vi "read numarray, compare with original one.vi"(0 "JSON in":string, 1 "binary data in":u8[](array[numeric]), 5 "array as variant in":variant, 7 "numeric type":T1, 9 "kwarg_name":string, 11 "error in (no error)":errorcluster, 12 "dims":u8) -> (3 "numarray 1D":cdb[](array[numeric]), 4 "numarray 2D":cdb[][](array[numeric]), 6 "numarray 3D":cdb[][][](array[numeric]), 8 "type out":dbl, 10 "arrays are equal":bool, 15 "error out":errorcluster)   [LabVIEW 2018, in "LV-Julia_ZMQ-Roundtrip_lib.lvlib"]
uses:
  LV-Julia_ZMQ-Roundtrip_lib.lvlib
  Numeric Types enum.ctl
  f90f2f60-c893-4d73-9894-bda48d86c5b6.vi
  1bcb8ed7-17cb-4152-8e47-ff7461b55bf4.vi
  05796eaf-ec06-43a6-a453-a404cbedcfeb.vi
  9b93abbe-6376-4f86-9348-90245d6e1835.vi
  760e0b37-cac3-4b4c-a236-19af47651068.vi
  729fa7d7-fd6d-49c0-b1c8-f0a08cd6f943.vi
  3b835e31-b93c-4e4c-9ac3-413a3184b071.vi
  5ec570e5-464f-4fa0-a09b-d89833ec3b5d.vi
  e2ab0a43-58c4-4b3b-8f56-301dfe696cbe.vi
  7bf60a27-5564-4d89-912b-dc8cfc55a1e3.vi
  6c204d97-3017-4fe4-991a-9f71cab6a49b.vi
  a9a31f31-ba5d-4a99-a09b-6ec61be075e6.vi
  2bab1b1a-04a3-4102-80c6-0860ef51feeb.vi
  f90f2f60-c893-4d73-9894-bda48d86c5b6.vi/aea26230-b37b-487e-9cf8-e6b3b36e77d0.vi
  f90f2f60-c893-4d73-9894-bda48d86c5b6.vi/eecf6d58-7644-48d9-827f-4c8cbdb10056.vi
  1bcb8ed7-17cb-4152-8e47-ff7461b55bf4.vi/d91edb37-e9cb-4de8-9c8b-37d9737b9146.vi
  1bcb8ed7-17cb-4152-8e47-ff7461b55bf4.vi/7f1f0db8-9b75-4073-a4d6-d2d0fba88da7.vi
  05796eaf-ec06-43a6-a453-a404cbedcfeb.vi/ae3ef386-b1b9-47a7-9bbe-131bd25933dd.vi
  05796eaf-ec06-43a6-a453-a404cbedcfeb.vi/d1185112-1ee5-44f5-9af4-afa5e2d7b356.vi
  9b93abbe-6376-4f86-9348-90245d6e1835.vi/4180a33d-dc17-4d50-82c8-ace037852335.vi
  9b93abbe-6376-4f86-9348-90245d6e1835.vi/eafb08bf-b040-4e13-8193-389eb035d60c.vi
  760e0b37-cac3-4b4c-a236-19af47651068.vi/44f6d320-ae0c-4b66-9297-4b8eca6fd43f.vi
  760e0b37-cac3-4b4c-a236-19af47651068.vi/0e4e9d1a-4190-4474-bb55-68a46c160070.vi
  729fa7d7-fd6d-49c0-b1c8-f0a08cd6f943.vi/3ce3e3bb-078a-4ec9-9189-4e9af33a938d.vi
  729fa7d7-fd6d-49c0-b1c8-f0a08cd6f943.vi/58c4dbd9-2697-4941-b5e4-ebe99b99620d.vi
  3b835e31-b93c-4e4c-9ac3-413a3184b071.vi/250f2895-05ca-44e8-b504-1634b1d2b405.vi
  3b835e31-b93c-4e4c-9ac3-413a3184b071.vi/e3331c0b-5588-4aa4-b191-8cdfd01c78f4.vi
  5ec570e5-464f-4fa0-a09b-d89833ec3b5d.vi/0062a4b9-4e16-4d04-a955-aedcc838ee20.vi
  5ec570e5-464f-4fa0-a09b-d89833ec3b5d.vi/d3ac89e5-0cbc-41e4-a6cb-834d9cdee77e.vi
  e2ab0a43-58c4-4b3b-8f56-301dfe696cbe.vi/ffe59d12-cb9c-4181-a501-418c11d92803.vi
  e2ab0a43-58c4-4b3b-8f56-301dfe696cbe.vi/ae3747c3-bc59-4fd4-b410-049d5a6f0db8.vi
  7bf60a27-5564-4d89-912b-dc8cfc55a1e3.vi/9fbfff10-2239-457d-9782-62788f7005e2.vi
  7bf60a27-5564-4d89-912b-dc8cfc55a1e3.vi/a3f15e31-3d6f-494d-b416-3d01e5211b04.vi
  6c204d97-3017-4fe4-991a-9f71cab6a49b.vi/b2b21668-f640-4c2e-a0b5-530a405b957c.vi
  6c204d97-3017-4fe4-991a-9f71cab6a49b.vi/329f9097-ea33-4282-b7c4-b8729ecdcad9.vi
  a9a31f31-ba5d-4a99-a09b-6ec61be075e6.vi/872a3bf9-871d-41eb-a9d3-de47e124106b.vi
  a9a31f31-ba5d-4a99-a09b-6ec61be075e6.vi/aa307742-699e-477b-9ebd-7d33a8d1c4a7.vi
  2bab1b1a-04a3-4102-80c6-0860ef51feeb.vi/accfd3bc-8c5f-419c-8a2f-c040c3b7ca9b.vi
  2bab1b1a-04a3-4102-80c6-0860ef51feeb.vi/ba93753e-6e06-4536-8801-a98345468d45.vi
  f90f2f60-c893-4d73-9894-bda48d86c5b6.vi/aea26230-b37b-487e-9cf8-e6b3b36e77d0.vi/3c276e99-f769-403a-993e-6bceeea52731.vi
  f90f2f60-c893-4d73-9894-bda48d86c5b6.vi/aea26230-b37b-487e-9cf8-e6b3b36e77d0.vi/085da6a5-152e-455b-bf9d-f293282960b1.vi
  1bcb8ed7-17cb-4152-8e47-ff7461b55bf4.vi/d91edb37-e9cb-4de8-9c8b-37d9737b9146.vi/c529b78e-4c21-4eee-bfac-2c8da8555f49.vi
  1bcb8ed7-17cb-4152-8e47-ff7461b55bf4.vi/d91edb37-e9cb-4de8-9c8b-37d9737b9146.vi/e59933f2-314b-4b4f-8e5f-2abbaebb5390.vi
  05796eaf-ec06-43a6-a453-a404cbedcfeb.vi/ae3ef386-b1b9-47a7-9bbe-131bd25933dd.vi/353adf82-e87c-4ddf-857a-0c8cbe8703d8.vi
  05796eaf-ec06-43a6-a453-a404cbedcfeb.vi/ae3ef386-b1b9-47a7-9bbe-131bd25933dd.vi/147a2d67-995c-467c-9951-50e059367510.vi
  9b93abbe-6376-4f86-9348-90245d6e1835.vi/4180a33d-dc17-4d50-82c8-ace037852335.vi/a812f023-13fb-4f61-8d22-99e25be0a908.vi
  9b93abbe-6376-4f86-9348-90245d6e1835.vi/4180a33d-dc17-4d50-82c8-ace037852335.vi/c7c0c08b-8ae7-4a4e-82ab-939504823c11.vi
  760e0b37-cac3-4b4c-a236-19af47651068.vi/44f6d320-ae0c-4b66-9297-4b8eca6fd43f.vi/c84abaef-c7ce-4c44-a01e-0d33354fe3f1.vi
  760e0b37-cac3-4b4c-a236-19af47651068.vi/44f6d320-ae0c-4b66-9297-4b8eca6fd43f.vi/6dbc9b59-227b-46ee-b802-76a43ccc2138.vi
  729fa7d7-fd6d-49c0-b1c8-f0a08cd6f943.vi/3ce3e3bb-078a-4ec9-9189-4e9af33a938d.vi/f6a97388-78b7-4eb1-a407-ba66989f46a1.vi
  729fa7d7-fd6d-49c0-b1c8-f0a08cd6f943.vi/3ce3e3bb-078a-4ec9-9189-4e9af33a938d.vi/c3509ff3-f9e7-4e3f-80ef-8fab03eb739a.vi
  3b835e31-b93c-4e4c-9ac3-413a3184b071.vi/250f2895-05ca-44e8-b504-1634b1d2b405.vi/624ddf69-388b-41f1-9bc3-bf65733aca34.vi
  3b835e31-b93c-4e4c-9ac3-413a3184b071.vi/250f2895-05ca-44e8-b504-1634b1d2b405.vi/a209ce17-74f1-4e04-9a76-a7e5c23822df.vi
  5ec570e5-464f-4fa0-a09b-d89833ec3b5d.vi/0062a4b9-4e16-4d04-a955-aedcc838ee20.vi/d12973b7-5bae-4b6c-8988-914ce2922173.vi
  5ec570e5-464f-4fa0-a09b-d89833ec3b5d.vi/0062a4b9-4e16-4d04-a955-aedcc838ee20.vi/e222edb4-4d07-4de1-833d-69e637ca4993.vi
  e2ab0a43-58c4-4b3b-8f56-301dfe696cbe.vi/ffe59d12-cb9c-4181-a501-418c11d92803.vi/c8694f25-7f4e-47d0-98e2-b06e60149a9d.vi
  e2ab0a43-58c4-4b3b-8f56-301dfe696cbe.vi/ffe59d12-cb9c-4181-a501-418c11d92803.vi/f32f3cf5-cc44-48b2-884a-30040af8c5d1.vi
  7bf60a27-5564-4d89-912b-dc8cfc55a1e3.vi/9fbfff10-2239-457d-9782-62788f7005e2.vi/faf29b4b-2bda-4a8a-b2e6-6da317472d00.vi
  7bf60a27-5564-4d89-912b-dc8cfc55a1e3.vi/9fbfff10-2239-457d-9782-62788f7005e2.vi/4a761303-963c-4ce3-9205-143dc320e55f.vi
  6c204d97-3017-4fe4-991a-9f71cab6a49b.vi/b2b21668-f640-4c2e-a0b5-530a405b957c.vi/3777e906-f595-4b33-903c-a1f5f2fb95d5.vi
  6c204d97-3017-4fe4-991a-9f71cab6a49b.vi/b2b21668-f640-4c2e-a0b5-530a405b957c.vi/0dc015e5-9aa0-46f4-a653-d68428c4d32a.vi
  a9a31f31-ba5d-4a99-a09b-6ec61be075e6.vi/872a3bf9-871d-41eb-a9d3-de47e124106b.vi/e5c3e3c4-ad55-4cee-8ec5-bc8269961401.vi
  a9a31f31-ba5d-4a99-a09b-6ec61be075e6.vi/872a3bf9-871d-41eb-a9d3-de47e124106b.vi/39b58c01-a45e-4308-8adf-eadd1e5539be.vi
  2bab1b1a-04a3-4102-80c6-0860ef51feeb.vi/accfd3bc-8c5f-419c-8a2f-c040c3b7ca9b.vi/10323f32-4176-42ce-b49d-47c887fd7cce.vi
  2bab1b1a-04a3-4102-80c6-0860ef51feeb.vi/accfd3bc-8c5f-419c-8a2f-c040c3b7ca9b.vi/c175c9d4-56ba-4ff5-b4b5-980da2c33c2a.vi
  f90f2f60-c893-4d73-9894-bda48d86c5b6.vi/aea26230-b37b-487e-9cf8-e6b3b36e77d0.vi/3c276e99-f769-403a-993e-6bceeea52731.vi/607607e7-0e9a-4aa0-9dec-04c7260ece5b.vi
  1bcb8ed7-17cb-4152-8e47-ff7461b55bf4.vi/d91edb37-e9cb-4de8-9c8b-37d9737b9146.vi/c529b78e-4c21-4eee-bfac-2c8da8555f49.vi/b19a4024-2a13-46f3-b1e6-4e15f4d8b153.vi
  05796eaf-ec06-43a6-a453-a404cbedcfeb.vi/ae3ef386-b1b9-47a7-9bbe-131bd25933dd.vi/353adf82-e87c-4ddf-857a-0c8cbe8703d8.vi/820e091e-b0e9-4f31-b0b9-e292fb03d7bf.vi
  9b93abbe-6376-4f86-9348-90245d6e1835.vi/4180a33d-dc17-4d50-82c8-ace037852335.vi/a812f023-13fb-4f61-8d22-99e25be0a908.vi/2ababed6-cce5-4a2c-adbf-e8086f6d75aa.vi
  760e0b37-cac3-4b4c-a236-19af47651068.vi/44f6d320-ae0c-4b66-9297-4b8eca6fd43f.vi/c84abaef-c7ce-4c44-a01e-0d33354fe3f1.vi/60c490a7-9a18-45a3-a996-e5a53239fa5d.vi
  729fa7d7-fd6d-49c0-b1c8-f0a08cd6f943.vi/3ce3e3bb-078a-4ec9-9189-4e9af33a938d.vi/f6a97388-78b7-4eb1-a407-ba66989f46a1.vi/c2c6e77e-694c-4a93-a97a-65d8b22958b3.vi
  3b835e31-b93c-4e4c-9ac3-413a3184b071.vi/250f2895-05ca-44e8-b504-1634b1d2b405.vi/624ddf69-388b-41f1-9bc3-bf65733aca34.vi/9e6dbe43-6f74-4f89-a3b9-2c6b8bd6acd4.vi
  5ec570e5-464f-4fa0-a09b-d89833ec3b5d.vi/0062a4b9-4e16-4d04-a955-aedcc838ee20.vi/d12973b7-5bae-4b6c-8988-914ce2922173.vi/dcfe2317-15ad-41a2-8b03-a5364eca9961.vi
  e2ab0a43-58c4-4b3b-8f56-301dfe696cbe.vi/ffe59d12-cb9c-4181-a501-418c11d92803.vi/c8694f25-7f4e-47d0-98e2-b06e60149a9d.vi/7fc37cc2-e941-4f9f-ba0c-fd92faf2991f.vi
  7bf60a27-5564-4d89-912b-dc8cfc55a1e3.vi/9fbfff10-2239-457d-9782-62788f7005e2.vi/faf29b4b-2bda-4a8a-b2e6-6da317472d00.vi/2da98f2e-d82c-46f1-9d88-f4916dfa7054.vi
  6c204d97-3017-4fe4-991a-9f71cab6a49b.vi/b2b21668-f640-4c2e-a0b5-530a405b957c.vi/3777e906-f595-4b33-903c-a1f5f2fb95d5.vi/010f70ef-59dc-4c7d-aa6c-1914130e20f9.vi
  a9a31f31-ba5d-4a99-a09b-6ec61be075e6.vi/872a3bf9-871d-41eb-a9d3-de47e124106b.vi/e5c3e3c4-ad55-4cee-8ec5-bc8269961401.vi/f4a1675d-9282-4ee1-a4cc-388fd1e856e9.vi
  <vilib>/Utility/error.llb/Error Cluster From Error Code.vi
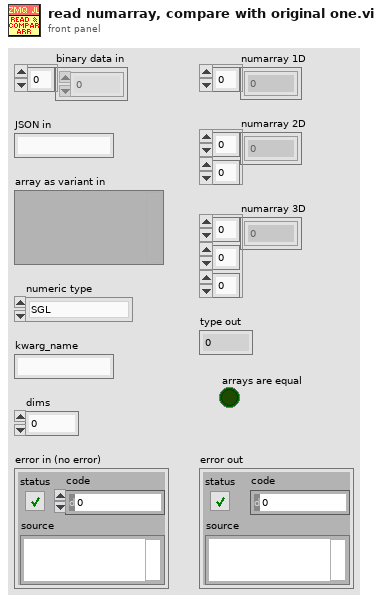
[diagram p1: front panel]
types:
  T1 = typedef "LV-Julia_ZMQ-Roundtrip_lib.lvlib/Numeric Types enum.ctl" = enum16{"SGL", "DBL", "I8", "I16", "I32", "I64", "U8", "U16", "U32", "U64", "CSGL", "CDBL", "boolean"}
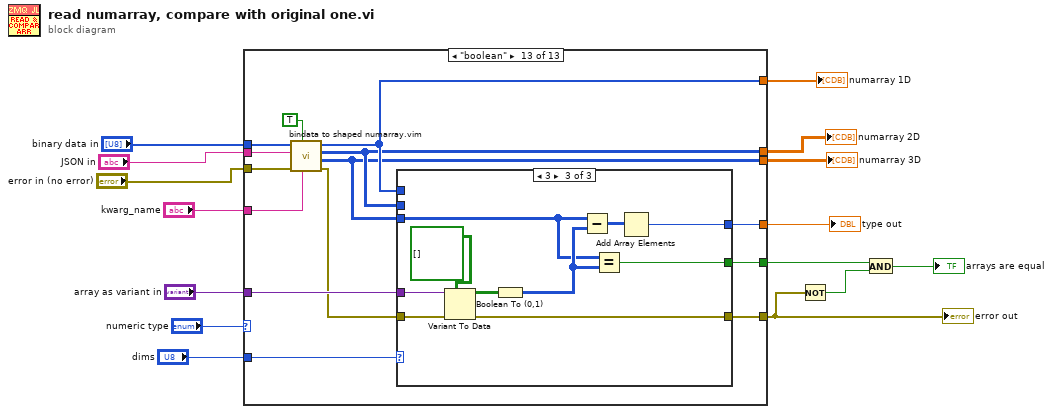
[diagram p0: block diagram]
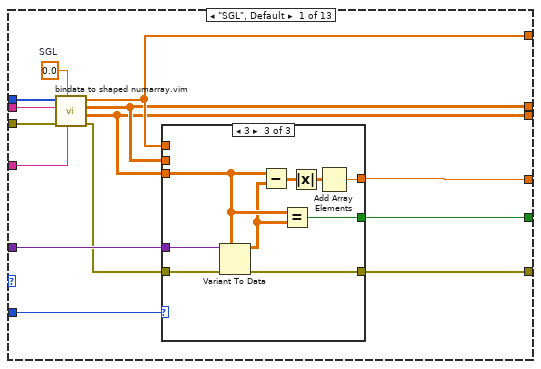
[diagram p2: hidden frame]
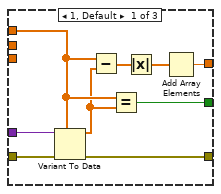
[diagram p3: hidden frame]
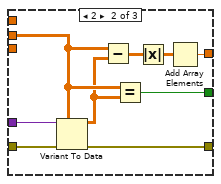
[diagram p4: hidden frame]
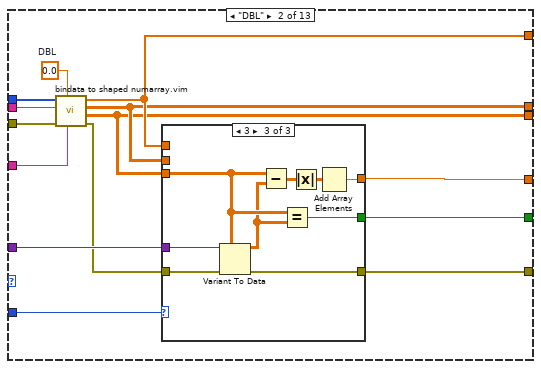
[diagram p5: hidden frame]
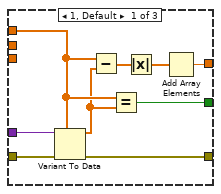
[diagram p6: hidden frame]
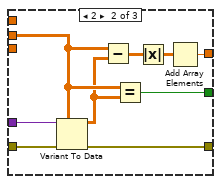
[diagram p7: hidden frame]
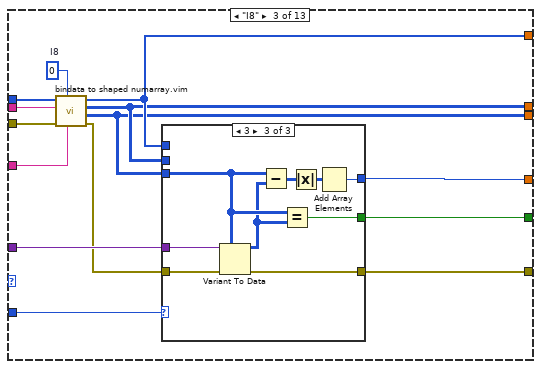
[diagram p8: hidden frame]
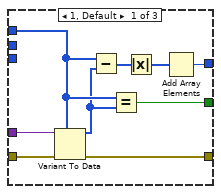
[diagram p9: hidden frame]
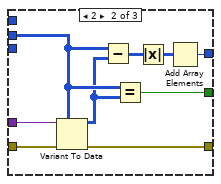
[diagram p10: hidden frame]
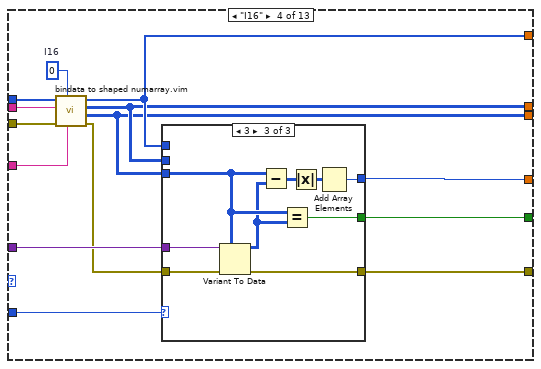
[diagram p11: hidden frame]
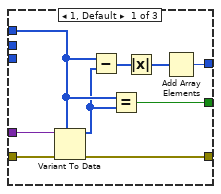
[diagram p12: hidden frame]
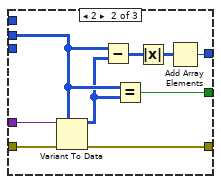
[diagram p13: hidden frame]
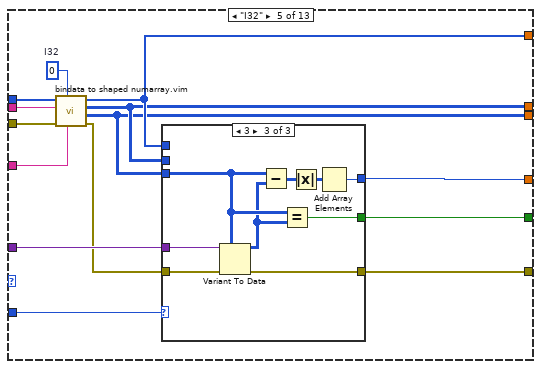
[diagram p14: hidden frame]
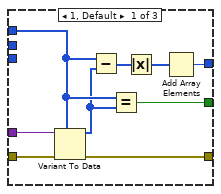
[diagram p15: hidden frame]
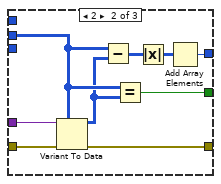
[diagram p16: hidden frame]
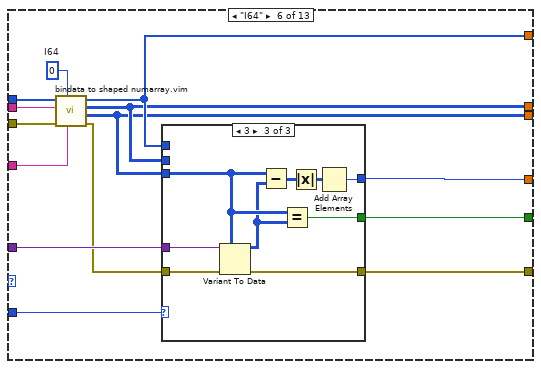
[diagram p17: hidden frame]
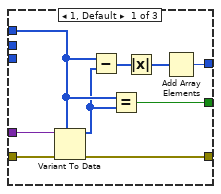
[diagram p18: hidden frame]
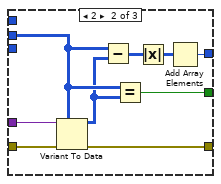
[diagram p19: hidden frame]
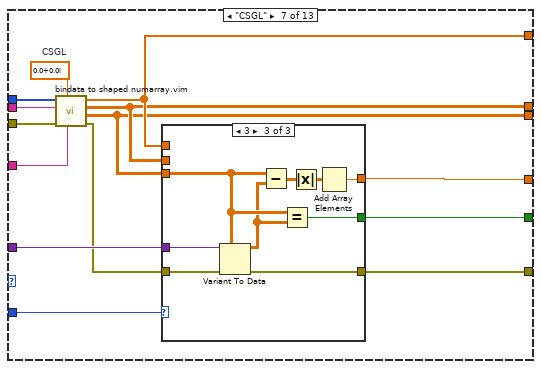
[diagram p20: hidden frame]
diagram:
  n1 = case shown="\"boolean\"" "numeric type" {
    tunnel: "error in (no error)" -> [w29 w70 w111 w152 w193 w234 w275 w316 w357 w395 w433 w471 w509]
    tunnel: "kwarg_name" -> [w28 w69 w110 w151 w192 w233 w274 w315 w356 w394 w432 w470 w508]
    tunnel: "binary data in" -> [w27 w68 w109 w150 w191 w232 w273 w314 w355 w393 w431 w469 w507]
    tunnel: "JSON in" -> [w26 w67 w108 w149 w190 w231 w272 w313 w354 w392 w430 w468 w506]
    tunnel: "dims" -> [w25 w66 w107 w148 w189 w230 w271 w312 w353 w391 w429 w467 w505]
    tunnel: [w24 w65 w106 w147 w188 w229 w270 w311 w352 w390 w428 w466 w504] -> w7
    tunnel: [w23 w64 w105 w146 w187 w228 w269 w310 w351 w389 w427 w465 w503] -> w8
    tunnel: [w22 w63 w104 w145 w186 w227 w268 w309 w350 w388 w426 w464 w502] -> w9
    tunnel: "array as variant in" -> [w21 w62 w103 w144 w185 w226 w267 w308 w349 w387 w425 w463 w501]
    tunnel: [w20 w61 w102 w143 w184 w225 w266 w307 w348 w386 w424 w462 w500] -> w2
    tunnel: [w19 w60 w101 w142 w183 w224 w265 w306 w347 w385 w423 w461 w499] -> w11
    tunnel: [w16 w57 w98 w139 w180 w221 w262 w303 w344 w382 w420 w458 w497] -> w12
    frame "SGL", Default {
      w17 = sgl 0.0  # SGL
      n2 = call "bindata to shaped numarray.vim"("kwarg_name"=w28, "data type"=w17, "error in (no error)"=w29, "bindata_descr"=w26, "binary data"=w27) -> ("error out"=w18:errorcluster, "numarray 3D"=w19:sgl[][][], "numarray 2D"=w23:sgl[][], "numarray 1D"=w24:sgl[])  [unwired: 3 in]
      n3 = case shown="3" w25 {
        tunnel: w24 -> [w32 _ _]
        tunnel: [w36 w45 w54] -> w22
        tunnel: w23 -> [_ w41 _]
        tunnel: w21 -> [w35 w44 w53]
        tunnel: w18 -> [w34 w43 w52]
        tunnel: [w33 w42 w51] -> w20
        tunnel: w19 -> [_ _ w50]
        tunnel: [w30 w39 w48] -> w16
        frame 1, Default {
          n4 = Variant To Data(error in=w34, type=w32, Variant=w35) -> (data=w31:sgl[], error out=w33:errorcluster)
          n5 = Subtract(x=w32, y=w31) -> (x-y=w38:sgl[])
          n6 = Equal?(x=w32, y=w31) -> (x = y?=w30:bool)
          n7 = Absolute Value(x=w38) -> (abs(x)=w37:sgl[])
          n8 = Add Array Elements(numeric array=w37) -> (sum=w36:sgl)
        }
        frame 2 {
          n9 = Variant To Data(error in=w43, type=w41, Variant=w44) -> (data=w40:sgl[][], error out=w42:errorcluster)
          n10 = Subtract(x=w41, y=w40) -> (x-y=w47:sgl[][])
          n11 = Equal?(x=w41, y=w40) -> (x = y?=w39:bool)
          n12 = Absolute Value(x=w47) -> (abs(x)=w46:sgl[][])
          n13 = Add Array Elements(numeric array=w46) -> (sum=w45:sgl)
        }
        frame 3 {
          n14 = Variant To Data(error in=w52, type=w50, Variant=w53) -> (data=w49:sgl[][][], error out=w51:errorcluster)
          n15 = Subtract(x=w50, y=w49) -> (x-y=w56:sgl[][][])
          n16 = Equal?(x=w50, y=w49) -> (x = y?=w48:bool)
          n17 = Absolute Value(x=w56) -> (abs(x)=w55:sgl[][][])
          n18 = Add Array Elements(numeric array=w55) -> (sum=w54:sgl)
        }
      }
    }
    frame "DBL" {
      w58 = 0.0  # DBL
      n19 = call "bindata to shaped numarray.vim"("kwarg_name"=w69, "data type"=w58, "error in (no error)"=w70, "bindata_descr"=w67, "binary data"=w68) -> ("error out"=w59:errorcluster, "numarray 3D"=w60:dbl[][][], "numarray 2D"=w64:dbl[][], "numarray 1D"=w65:dbl[])  [unwired: 3 in]
      n20 = case shown="3" w66 {
        tunnel: w65 -> [w73 _ _]
        tunnel: [w77 w86 w95] -> w63
        tunnel: w64 -> [_ w82 _]
        tunnel: w62 -> [w76 w85 w94]
        tunnel: w59 -> [w75 w84 w93]
        tunnel: [w74 w83 w92] -> w61
        tunnel: w60 -> [_ _ w91]
        tunnel: [w71 w80 w89] -> w57
        frame 1, Default {
          n21 = Variant To Data(error in=w75, type=w73, Variant=w76) -> (data=w72:dbl[], error out=w74:errorcluster)
          n22 = Subtract(x=w73, y=w72) -> (x-y=w79:dbl[])
          n23 = Equal?(x=w73, y=w72) -> (x = y?=w71:bool)
          n24 = Absolute Value(x=w79) -> (abs(x)=w78:dbl[])
          n25 = Add Array Elements(numeric array=w78) -> (sum=w77:dbl)
        }
        frame 2 {
          n26 = Variant To Data(error in=w84, type=w82, Variant=w85) -> (data=w81:dbl[][], error out=w83:errorcluster)
          n27 = Subtract(x=w82, y=w81) -> (x-y=w88:dbl[][])
          n28 = Equal?(x=w82, y=w81) -> (x = y?=w80:bool)
          n29 = Absolute Value(x=w88) -> (abs(x)=w87:dbl[][])
          n30 = Add Array Elements(numeric array=w87) -> (sum=w86:dbl)
        }
        frame 3 {
          n31 = Variant To Data(error in=w93, type=w91, Variant=w94) -> (data=w90:dbl[][][], error out=w92:errorcluster)
          n32 = Subtract(x=w91, y=w90) -> (x-y=w97:dbl[][][])
          n33 = Equal?(x=w91, y=w90) -> (x = y?=w89:bool)
          n34 = Absolute Value(x=w97) -> (abs(x)=w96:dbl[][][])
          n35 = Add Array Elements(numeric array=w96) -> (sum=w95:dbl)
        }
      }
    }
    frame "I8" {
      w99 = i8 0  # I8
      n36 = call "bindata to shaped numarray.vim"("kwarg_name"=w110, "data type"=w99, "error in (no error)"=w111, "bindata_descr"=w108, "binary data"=w109) -> ("error out"=w100:errorcluster, "numarray 3D"=w101:i8[][][], "numarray 2D"=w105:i8[][], "numarray 1D"=w106:i8[])  [unwired: 3 in]
      n37 = case shown="3" w107 {
        tunnel: w106 -> [w114 _ _]
        tunnel: [w118 w127 w136] -> w104
        tunnel: w105 -> [_ w123 _]
        tunnel: w103 -> [w117 w126 w135]
        tunnel: w100 -> [w116 w125 w134]
        tunnel: [w115 w124 w133] -> w102
        tunnel: w101 -> [_ _ w132]
        tunnel: [w112 w121 w130] -> w98
        frame 1, Default {
          n38 = Variant To Data(error in=w116, type=w114, Variant=w117) -> (data=w113:i8[], error out=w115:errorcluster)
          n39 = Subtract(x=w114, y=w113) -> (x-y=w120:i8[])
          n40 = Equal?(x=w114, y=w113) -> (x = y?=w112:bool)
          n41 = Absolute Value(x=w120) -> (abs(x)=w119:i8[])
          n42 = Add Array Elements(numeric array=w119) -> (sum=w118:i8)
        }
        frame 2 {
          n43 = Variant To Data(error in=w125, type=w123, Variant=w126) -> (data=w122:i8[][], error out=w124:errorcluster)
          n44 = Subtract(x=w123, y=w122) -> (x-y=w129:i8[][])
          n45 = Equal?(x=w123, y=w122) -> (x = y?=w121:bool)
          n46 = Absolute Value(x=w129) -> (abs(x)=w128:i8[][])
          n47 = Add Array Elements(numeric array=w128) -> (sum=w127:i8)
        }
        frame 3 {
          n48 = Variant To Data(error in=w134, type=w132, Variant=w135) -> (data=w131:i8[][][], error out=w133:errorcluster)
          n49 = Subtract(x=w132, y=w131) -> (x-y=w138:i8[][][])
          n50 = Equal?(x=w132, y=w131) -> (x = y?=w130:bool)
          n51 = Absolute Value(x=w138) -> (abs(x)=w137:i8[][][])
          n52 = Add Array Elements(numeric array=w137) -> (sum=w136:i8)
        }
      }
    }
    frame "I16" {
      w140 = i16 0  # I16
      n53 = call "bindata to shaped numarray.vim"("kwarg_name"=w151, "data type"=w140, "error in (no error)"=w152, "bindata_descr"=w149, "binary data"=w150) -> ("error out"=w141:errorcluster, "numarray 3D"=w142:i16[][][], "numarray 2D"=w146:i16[][], "numarray 1D"=w147:i16[])  [unwired: 3 in]
      n54 = case shown="3" w148 {
        tunnel: w147 -> [w155 _ _]
        tunnel: [w159 w168 w177] -> w145
        tunnel: w146 -> [_ w164 _]
        tunnel: w144 -> [w158 w167 w176]
        tunnel: w141 -> [w157 w166 w175]
        tunnel: [w156 w165 w174] -> w143
        tunnel: w142 -> [_ _ w173]
        tunnel: [w153 w162 w171] -> w139
        frame 1, Default {
          n55 = Variant To Data(error in=w157, type=w155, Variant=w158) -> (data=w154:i16[], error out=w156:errorcluster)
          n56 = Subtract(x=w155, y=w154) -> (x-y=w161:i16[])
          n57 = Equal?(x=w155, y=w154) -> (x = y?=w153:bool)
          n58 = Absolute Value(x=w161) -> (abs(x)=w160:i16[])
          n59 = Add Array Elements(numeric array=w160) -> (sum=w159:i16)
        }
        frame 2 {
          n60 = Variant To Data(error in=w166, type=w164, Variant=w167) -> (data=w163:i16[][], error out=w165:errorcluster)
          n61 = Subtract(x=w164, y=w163) -> (x-y=w170:i16[][])
          n62 = Equal?(x=w164, y=w163) -> (x = y?=w162:bool)
          n63 = Absolute Value(x=w170) -> (abs(x)=w169:i16[][])
          n64 = Add Array Elements(numeric array=w169) -> (sum=w168:i16)
        }
        frame 3 {
          n65 = Variant To Data(error in=w175, type=w173, Variant=w176) -> (data=w172:i16[][][], error out=w174:errorcluster)
          n66 = Subtract(x=w173, y=w172) -> (x-y=w179:i16[][][])
          n67 = Equal?(x=w173, y=w172) -> (x = y?=w171:bool)
          n68 = Absolute Value(x=w179) -> (abs(x)=w178:i16[][][])
          n69 = Add Array Elements(numeric array=w178) -> (sum=w177:i16)
        }
      }
    }
    frame "I32" {
      w181 = 0  # I32
      n70 = call "bindata to shaped numarray.vim"("kwarg_name"=w192, "data type"=w181, "error in (no error)"=w193, "bindata_descr"=w190, "binary data"=w191) -> ("error out"=w182:errorcluster, "numarray 3D"=w183:i32[][][], "numarray 2D"=w187:i32[][], "numarray 1D"=w188:i32[])  [unwired: 3 in]
      n71 = case shown="3" w189 {
        tunnel: w188 -> [w196 _ _]
        tunnel: [w200 w209 w218] -> w186
        tunnel: w187 -> [_ w205 _]
        tunnel: w185 -> [w199 w208 w217]
        tunnel: w182 -> [w198 w207 w216]
        tunnel: [w197 w206 w215] -> w184
        tunnel: w183 -> [_ _ w214]
        tunnel: [w194 w203 w212] -> w180
        frame 1, Default {
          n72 = Variant To Data(error in=w198, type=w196, Variant=w199) -> (data=w195:i32[], error out=w197:errorcluster)
          n73 = Subtract(x=w196, y=w195) -> (x-y=w202:i32[])
          n74 = Equal?(x=w196, y=w195) -> (x = y?=w194:bool)
          n75 = Absolute Value(x=w202) -> (abs(x)=w201:i32[])
          n76 = Add Array Elements(numeric array=w201) -> (sum=w200:i32)
        }
        frame 2 {
          n77 = Variant To Data(error in=w207, type=w205, Variant=w208) -> (data=w204:i32[][], error out=w206:errorcluster)
          n78 = Subtract(x=w205, y=w204) -> (x-y=w211:i32[][])
          n79 = Equal?(x=w205, y=w204) -> (x = y?=w203:bool)
          n80 = Absolute Value(x=w211) -> (abs(x)=w210:i32[][])
          n81 = Add Array Elements(numeric array=w210) -> (sum=w209:i32)
        }
        frame 3 {
          n82 = Variant To Data(error in=w216, type=w214, Variant=w217) -> (data=w213:i32[][][], error out=w215:errorcluster)
          n83 = Subtract(x=w214, y=w213) -> (x-y=w220:i32[][][])
          n84 = Equal?(x=w214, y=w213) -> (x = y?=w212:bool)
          n85 = Absolute Value(x=w220) -> (abs(x)=w219:i32[][][])
          n86 = Add Array Elements(numeric array=w219) -> (sum=w218:i32)
        }
      }
    }
    frame "I64" {
      w222 = i64 0  # I64
      n87 = call "bindata to shaped numarray.vim"("kwarg_name"=w233, "data type"=w222, "error in (no error)"=w234, "bindata_descr"=w231, "binary data"=w232) -> ("error out"=w223:errorcluster, "numarray 3D"=w224:i64[][][], "numarray 2D"=w228:i64[][], "numarray 1D"=w229:i64[])  [unwired: 3 in]
      n88 = case shown="3" w230 {
        tunnel: w229 -> [w237 _ _]
        tunnel: [w241 w250 w259] -> w227
        tunnel: w228 -> [_ w246 _]
        tunnel: w226 -> [w240 w249 w258]
        tunnel: w223 -> [w239 w248 w257]
        tunnel: [w238 w247 w256] -> w225
        tunnel: w224 -> [_ _ w255]
        tunnel: [w235 w244 w253] -> w221
        frame 1, Default {
          n89 = Variant To Data(error in=w239, type=w237, Variant=w240) -> (data=w236:i64[], error out=w238:errorcluster)
          n90 = Subtract(x=w237, y=w236) -> (x-y=w243:i64[])
          n91 = Equal?(x=w237, y=w236) -> (x = y?=w235:bool)
          n92 = Absolute Value(x=w243) -> (abs(x)=w242:i64[])
          n93 = Add Array Elements(numeric array=w242) -> (sum=w241:i64)
        }
        frame 2 {
          n94 = Variant To Data(error in=w248, type=w246, Variant=w249) -> (data=w245:i64[][], error out=w247:errorcluster)
          n95 = Subtract(x=w246, y=w245) -> (x-y=w252:i64[][])
          n96 = Equal?(x=w246, y=w245) -> (x = y?=w244:bool)
          n97 = Absolute Value(x=w252) -> (abs(x)=w251:i64[][])
          n98 = Add Array Elements(numeric array=w251) -> (sum=w250:i64)
        }
        frame 3 {
          n99 = Variant To Data(error in=w257, type=w255, Variant=w258) -> (data=w254:i64[][][], error out=w256:errorcluster)
          n100 = Subtract(x=w255, y=w254) -> (x-y=w261:i64[][][])
          n101 = Equal?(x=w255, y=w254) -> (x = y?=w253:bool)
          n102 = Absolute Value(x=w261) -> (abs(x)=w260:i64[][][])
          n103 = Add Array Elements(numeric array=w260) -> (sum=w259:i64)
        }
      }
    }
    frame "CSGL" {
      w263 = csg 0.0+0.0i  # CSGL
      n104 = call "bindata to shaped numarray.vim"("kwarg_name"=w274, "data type"=w263, "error in (no error)"=w275, "bindata_descr"=w272, "binary data"=w273) -> ("error out"=w264:errorcluster, "numarray 3D"=w265:csg[][][], "numarray 2D"=w269:csg[][], "numarray 1D"=w270:csg[])  [unwired: 3 in]
      n105 = case shown="3" w271 {
        tunnel: w270 -> [w278 _ _]
        tunnel: [w282 w291 w300] -> w268
        tunnel: w269 -> [_ w287 _]
        tunnel: w267 -> [w281 w290 w299]
        tunnel: w264 -> [w280 w289 w298]
        tunnel: [w279 w288 w297] -> w266
        tunnel: w265 -> [_ _ w296]
        tunnel: [w276 w285 w294] -> w262
        frame 1, Default {
          n106 = Variant To Data(error in=w280, type=w278, Variant=w281) -> (data=w277:csg[], error out=w279:errorcluster)
          n107 = Subtract(x=w278, y=w277) -> (x-y=w284:csg[])
          n108 = Equal?(x=w278, y=w277) -> (x = y?=w276:bool)
          n109 = Absolute Value(x=w284) -> (abs(x)=w283:sgl[])
          n110 = Add Array Elements(numeric array=w283) -> (sum=w282:sgl)
        }
        frame 2 {
          n111 = Variant To Data(error in=w289, type=w287, Variant=w290) -> (data=w286:csg[][], error out=w288:errorcluster)
          n112 = Subtract(x=w287, y=w286) -> (x-y=w293:csg[][])
          n113 = Equal?(x=w287, y=w286) -> (x = y?=w285:bool)
          n114 = Absolute Value(x=w293) -> (abs(x)=w292:sgl[][])
          n115 = Add Array Elements(numeric array=w292) -> (sum=w291:sgl)
        }
        frame 3 {
          n116 = Variant To Data(error in=w298, type=w296, Variant=w299) -> (data=w295:csg[][][], error out=w297:errorcluster)
          n117 = Subtract(x=w296, y=w295) -> (x-y=w302:csg[][][])
          n118 = Equal?(x=w296, y=w295) -> (x = y?=w294:bool)
          n119 = Absolute Value(x=w302) -> (abs(x)=w301:sgl[][][])
          n120 = Add Array Elements(numeric array=w301) -> (sum=w300:sgl)
        }
      }
    }
    frame "CDBL" {
      w304 = cdb 0.0+0.0i  # CDBL
      n121 = call "bindata to shaped numarray.vim"("kwarg_name"=w315, "data type"=w304, "error in (no error)"=w316, "bindata_descr"=w313, "binary data"=w314) -> ("error out"=w305:errorcluster, "numarray 3D"=w306:cdb[][][], "numarray 2D"=w310:cdb[][], "numarray 1D"=w311:cdb[])  [unwired: 3 in]
      n122 = case shown="3" w312 {
        tunnel: w311 -> [w319 _ _]
        tunnel: [w323 w332 w341] -> w309
        tunnel: w310 -> [_ w328 _]
        tunnel: w308 -> [w322 w331 w340]
        tunnel: w305 -> [w321 w330 w339]
        tunnel: [w320 w329 w338] -> w307
        tunnel: w306 -> [_ _ w337]
        tunnel: [w317 w326 w335] -> w303
        frame 1, Default {
          n123 = Variant To Data(error in=w321, type=w319, Variant=w322) -> (data=w318:cdb[], error out=w320:errorcluster)
          n124 = Subtract(x=w319, y=w318) -> (x-y=w325:cdb[])
          n125 = Equal?(x=w319, y=w318) -> (x = y?=w317:bool)
          n126 = Absolute Value(x=w325) -> (abs(x)=w324:dbl[])
          n127 = Add Array Elements(numeric array=w324) -> (sum=w323:dbl)
        }
        frame 2 {
          n128 = Variant To Data(error in=w330, type=w328, Variant=w331) -> (data=w327:cdb[][], error out=w329:errorcluster)
          n129 = Subtract(x=w328, y=w327) -> (x-y=w334:cdb[][])
          n130 = Equal?(x=w328, y=w327) -> (x = y?=w326:bool)
          n131 = Absolute Value(x=w334) -> (abs(x)=w333:dbl[][])
          n132 = Add Array Elements(numeric array=w333) -> (sum=w332:dbl)
        }
        frame 3 {
          n133 = Variant To Data(error in=w339, type=w337, Variant=w340) -> (data=w336:cdb[][][], error out=w338:errorcluster)
          n134 = Subtract(x=w337, y=w336) -> (x-y=w343:cdb[][][])
          n135 = Equal?(x=w337, y=w336) -> (x = y?=w335:bool)
          n136 = Absolute Value(x=w343) -> (abs(x)=w342:dbl[][][])
          n137 = Add Array Elements(numeric array=w342) -> (sum=w341:dbl)
        }
      }
    }
    frame "U8" {
      w345 = u8 0  # U8
      n138 = call "bindata to shaped numarray.vim"("kwarg_name"=w356, "data type"=w345, "error in (no error)"=w357, "bindata_descr"=w354, "binary data"=w355) -> ("error out"=w346:errorcluster, "numarray 3D"=w347:u8[][][], "numarray 2D"=w351:u8[][], "numarray 1D"=w352:u8[])  [unwired: 3 in]
      n139 = case shown="2" w353 {
        tunnel: w352 -> [w361 _ _]
        tunnel: [w365 w373 w381] -> w350
        tunnel: w351 -> [_ w369 _]
        tunnel: w349 -> [w364 w372 w380]
        tunnel: w346 -> [w363 w371 w379]
        tunnel: [w362 w370 w378] -> w348
        tunnel: w347 -> [_ _ w377]
        tunnel: [w359 w367 w375] -> w344
        frame 1, Default {
          n140 = Variant To Data(error in=w363, type=w361, Variant=w364) -> (data=w360:u8[], error out=w362:errorcluster)
          n141 = Subtract(x=w361, y=w360) -> (x-y=w358:u8[])
          n142 = Equal?(x=w361, y=w360) -> (x = y?=w359:bool)
          n143 = Add Array Elements(numeric array=w358) -> (sum=w365:u8)
        }
        frame 2 {
          n144 = Variant To Data(error in=w371, type=w369, Variant=w372) -> (data=w368:u8[][], error out=w370:errorcluster)
          n145 = Subtract(x=w369, y=w368) -> (x-y=w366:u8[][])
          n146 = Equal?(x=w369, y=w368) -> (x = y?=w367:bool)
          n147 = Add Array Elements(numeric array=w366) -> (sum=w373:u8)
        }
        frame 3 {
          n148 = Variant To Data(error in=w379, type=w377, Variant=w380) -> (data=w376:u8[][][], error out=w378:errorcluster)
          n149 = Subtract(x=w377, y=w376) -> (x-y=w374:u8[][][])
          n150 = Equal?(x=w377, y=w376) -> (x = y?=w375:bool)
          n151 = Add Array Elements(numeric array=w374) -> (sum=w381:u8)
        }
      }
    }
    frame "U16" {
      w383 = u16 0  # U16
      n152 = call "bindata to shaped numarray.vim"("kwarg_name"=w394, "data type"=w383, "error in (no error)"=w395, "bindata_descr"=w392, "binary data"=w393) -> ("error out"=w384:errorcluster, "numarray 3D"=w385:u16[][][], "numarray 2D"=w389:u16[][], "numarray 1D"=w390:u16[])  [unwired: 3 in]
      n153 = case shown="2" w391 {
        tunnel: w390 -> [w399 _ _]
        tunnel: [w403 w411 w419] -> w388
        tunnel: w389 -> [_ w407 _]
        tunnel: w387 -> [w402 w410 w418]
        tunnel: w384 -> [w401 w409 w417]
        tunnel: [w400 w408 w416] -> w386
        tunnel: w385 -> [_ _ w415]
        tunnel: [w397 w405 w413] -> w382
        frame 1, Default {
          n154 = Variant To Data(error in=w401, type=w399, Variant=w402) -> (data=w398:u16[], error out=w400:errorcluster)
          n155 = Subtract(x=w399, y=w398) -> (x-y=w396:u16[])
          n156 = Equal?(x=w399, y=w398) -> (x = y?=w397:bool)
          n157 = Add Array Elements(numeric array=w396) -> (sum=w403:u16)
        }
        frame 2 {
          n158 = Variant To Data(error in=w409, type=w407, Variant=w410) -> (data=w406:u16[][], error out=w408:errorcluster)
          n159 = Subtract(x=w407, y=w406) -> (x-y=w404:u16[][])
          n160 = Equal?(x=w407, y=w406) -> (x = y?=w405:bool)
          n161 = Add Array Elements(numeric array=w404) -> (sum=w411:u16)
        }
        frame 3 {
          n162 = Variant To Data(error in=w417, type=w415, Variant=w418) -> (data=w414:u16[][][], error out=w416:errorcluster)
          n163 = Subtract(x=w415, y=w414) -> (x-y=w412:u16[][][])
          n164 = Equal?(x=w415, y=w414) -> (x = y?=w413:bool)
          n165 = Add Array Elements(numeric array=w412) -> (sum=w419:u16)
        }
      }
    }
    frame "U32" {
      w421 = u32 0  # U32
      n166 = call "bindata to shaped numarray.vim"("kwarg_name"=w432, "data type"=w421, "error in (no error)"=w433, "bindata_descr"=w430, "binary data"=w431) -> ("error out"=w422:errorcluster, "numarray 3D"=w423:u32[][][], "numarray 2D"=w427:u32[][], "numarray 1D"=w428:u32[])  [unwired: 3 in]
      n167 = case shown="2" w429 {
        tunnel: w428 -> [w437 _ _]
        tunnel: [w441 w449 w457] -> w426
        tunnel: w427 -> [_ w445 _]
        tunnel: w425 -> [w440 w448 w456]
        tunnel: w422 -> [w439 w447 w455]
        tunnel: [w438 w446 w454] -> w424
        tunnel: w423 -> [_ _ w453]
        tunnel: [w435 w443 w451] -> w420
        frame 1, Default {
          n168 = Variant To Data(error in=w439, type=w437, Variant=w440) -> (data=w436:u32[], error out=w438:errorcluster)
          n169 = Subtract(x=w437, y=w436) -> (x-y=w434:u32[])
          n170 = Equal?(x=w437, y=w436) -> (x = y?=w435:bool)
          n171 = Add Array Elements(numeric array=w434) -> (sum=w441:u32)
        }
        frame 2 {
          n172 = Variant To Data(error in=w447, type=w445, Variant=w448) -> (data=w444:u32[][], error out=w446:errorcluster)
          n173 = Subtract(x=w445, y=w444) -> (x-y=w442:u32[][])
          n174 = Equal?(x=w445, y=w444) -> (x = y?=w443:bool)
          n175 = Add Array Elements(numeric array=w442) -> (sum=w449:u32)
        }
        frame 3 {
          n176 = Variant To Data(error in=w455, type=w453, Variant=w456) -> (data=w452:u32[][][], error out=w454:errorcluster)
          n177 = Subtract(x=w453, y=w452) -> (x-y=w450:u32[][][])
          n178 = Equal?(x=w453, y=w452) -> (x = y?=w451:bool)
          n179 = Add Array Elements(numeric array=w450) -> (sum=w457:u32)
        }
      }
    }
    frame "U64" {
      w459 = u64 0  # U64
      n180 = call "bindata to shaped numarray.vim"("kwarg_name"=w470, "data type"=w459, "error in (no error)"=w471, "bindata_descr"=w468, "binary data"=w469) -> ("error out"=w460:errorcluster, "numarray 3D"=w461:u64[][][], "numarray 2D"=w465:u64[][], "numarray 1D"=w466:u64[])  [unwired: 3 in]
      n181 = case shown="2" w467 {
        tunnel: w466 -> [w475 _ _]
        tunnel: [w479 w487 w495] -> w464
        tunnel: w465 -> [_ w483 _]
        tunnel: w463 -> [w478 w486 w494]
        tunnel: w460 -> [w477 w485 w493]
        tunnel: [w476 w484 w492] -> w462
        tunnel: w461 -> [_ _ w491]
        tunnel: [w473 w481 w489] -> w458
        frame 1, Default {
          n182 = Variant To Data(error in=w477, type=w475, Variant=w478) -> (data=w474:u64[], error out=w476:errorcluster)
          n183 = Subtract(x=w475, y=w474) -> (x-y=w472:u64[])
          n184 = Equal?(x=w475, y=w474) -> (x = y?=w473:bool)
          n185 = Add Array Elements(numeric array=w472) -> (sum=w479:u64)
        }
        frame 2 {
          n186 = Variant To Data(error in=w485, type=w483, Variant=w486) -> (data=w482:u64[][], error out=w484:errorcluster)
          n187 = Subtract(x=w483, y=w482) -> (x-y=w480:u64[][])
          n188 = Equal?(x=w483, y=w482) -> (x = y?=w481:bool)
          n189 = Add Array Elements(numeric array=w480) -> (sum=w487:u64)
        }
        frame 3 {
          n190 = Variant To Data(error in=w493, type=w491, Variant=w494) -> (data=w490:u64[][][], error out=w492:errorcluster)
          n191 = Subtract(x=w491, y=w490) -> (x-y=w488:u64[][][])
          n192 = Equal?(x=w491, y=w490) -> (x = y?=w489:bool)
          n193 = Add Array Elements(numeric array=w488) -> (sum=w495:u64)
        }
      }
    }
    frame "boolean" {
      n194 = call "bindata to shaped numarray.vim"("kwarg_name"=w508, "data type"=TRUE, "error in (no error)"=w509, "bindata_descr"=w506, "binary data"=w507) -> ("error out"=w498:errorcluster, "numarray 3D"=w499:u8[][][], "numarray 2D"=w503:u8[][], "numarray 1D"=w504:u8[])  [unwired: 3 in]
      n195 = case shown="3" w505 {
        tunnel: w504 -> [w510 _ _]
        tunnel: [w519 w529 w539] -> w502
        tunnel: w503 -> [_ w525 _]
        tunnel: w501 -> [w518 w528 w538]
        tunnel: w498 -> [w517 w527 w537]
        tunnel: [w516 w526 w536] -> w500
        tunnel: w499 -> [_ _ w530]
        tunnel: [w514 w523 w534] -> w497
        frame 1, Default {
          n196 = Variant To Data(error in=w517, type=bool[] [], Variant=w518) -> (data=w515:bool[], error out=w516:errorcluster)
          n197 = Boolean To (0,1)(Boolean=w515) -> (0, 1=w511:i16[])
          n198 = Subtract(x=w510, y=w511) -> (x-y=w513:i16[])
          n199 = Equal?(x=w510, y=w511) -> (x = y?=w514:bool)
          n200 = Add Array Elements(numeric array=w513) -> (sum=w519:i16)
        }
        frame 2 {
          n201 = Variant To Data(error in=w527, type=bool[][] [], Variant=w528) -> (data=w524:bool[][], error out=w526:errorcluster)
          n202 = Boolean To (0,1)(Boolean=w524) -> (0, 1=w520:i16[][])
          n203 = Subtract(x=w525, y=w520) -> (x-y=w522:i16[][])
          n204 = Equal?(x=w525, y=w520) -> (x = y?=w523:bool)
          n205 = Add Array Elements(numeric array=w522) -> (sum=w529:i16)
        }
        frame 3 {
          n206 = Variant To Data(error in=w537, type=bool[][][] [], Variant=w538) -> (data=w535:bool[][][], error out=w536:errorcluster)
          n207 = Boolean To (0,1)(Boolean=w535) -> (0, 1=w531:i16[][][])
          n208 = Subtract(x=w530, y=w531) -> (x-y=w533:i16[][][])
          n209 = Equal?(x=w530, y=w531) -> (x = y?=w534:bool)
          n210 = Add Array Elements(numeric array=w533) -> (sum=w539:i16)
        }
      }
    }
  }
  "numarray 3D" <- w11
  "error out" <- w2
  "type out" <- w9
  "numarray 2D" <- w8
  "numarray 1D" <- w7
  n211 = Not(x=w2) -> (.not. x?=w1:bool)
  n212 = And(x=w12, y=w1) -> (x .and. y?=→"arrays are equal":bool)
